vi "Add Child Enqueuer.vi"(8 "error in (no error)":errorcluster, 10 "Nested Actor's Enqueuer":refnum<class "Message Enqueuer.lvclass">, 11 "RDS Root Actor in":refnum<class "RDS Root Actor.lvclass">) -> (0 "error out":errorcluster, 3 "RDS Root Actor out":refnum<class "RDS Root Actor.lvclass">)   [LabVIEW 2015, in "RDS Root Actor.lvlib" / "RDS Root Actor.lvclass"]
uses:
  RDS Root Actor.lvclass
  <vilib>/ActorFramework/Message Enqueuer/Message Enqueuer.lvclass
  RDS Root Actor.lvclass/RDS Root Actor.ctl
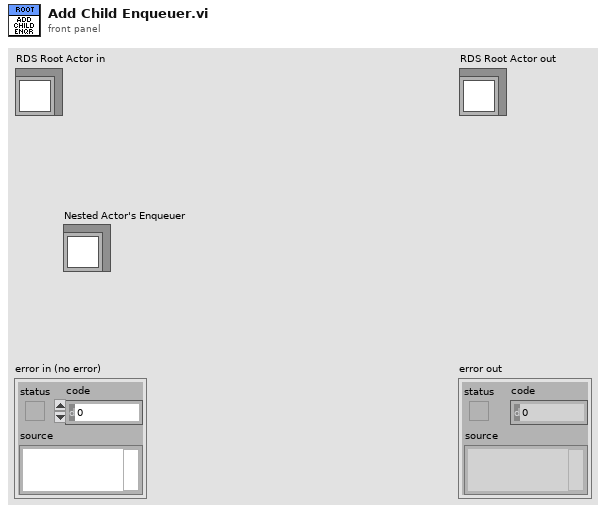
[diagram p1: front panel]
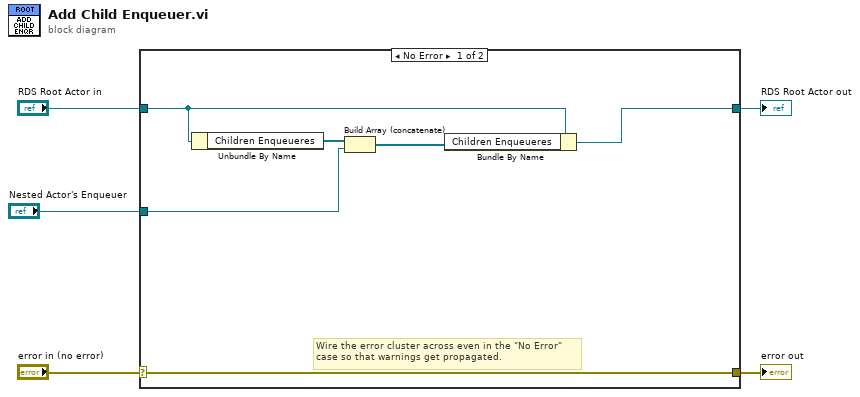
[diagram p0: block diagram]
diagram:
  n1 = case shown="No Error" "error in (no error)" {
    selector: "error in (no error)" -> [w11 w13]
    tunnel: [w11 w13] -> w4
    tunnel: [w6 w12] -> w2
    tunnel: "RDS Root Actor in" -> [w7 w12]
    tunnel: "Nested Actor's Enqueuer" -> [w9 _]
    frame No Error {
      # "Wire the error cluster across even in the \"No Error\"\ncase so that warnings get propagated."
      n2 = Unbundle By Name(w7) -> ("Children Enqueueres"=w10:refnum<class "Message Enqueuer.lvclass">[])
      n3 = Build Array (concatenate)(w10, w9) -> (w8:refnum<class "Message Enqueuer.lvclass">[])
      n4 = Bundle By Name(cluster=w7, "Children Enqueueres"=w8) -> (w6:refnum<class "RDS Root Actor.lvclass">)
    }
    frame Error {
    }
  }
  "error out" <- w4
  "RDS Root Actor out" <- w2
